vi "写入多个寄存器新.vi"(7 "VISA Resource":refnum<visa-resource-name>, 8 "Error in":errorcluster caption="Error in (no error)", 10 "values":u16[](array[numeric]), 11 "starting address":u16) -> (0 "error out":errorcluster)   [LabVIEW 2016, in "斯坦道CODMn.lvlib"]
uses:
  <vilib>/Plasmionique/MB Master/MB_Master_Serial/MB_Master_Serial.lvclass
  F:/Program Files/National Instruments/LabVIEW 2016/vi.lib/Plasmionique/MB Master/MB_Master/MB_Master.lvclass
  <vilib>/Plasmionique/MB Master/MB Master.lvlib
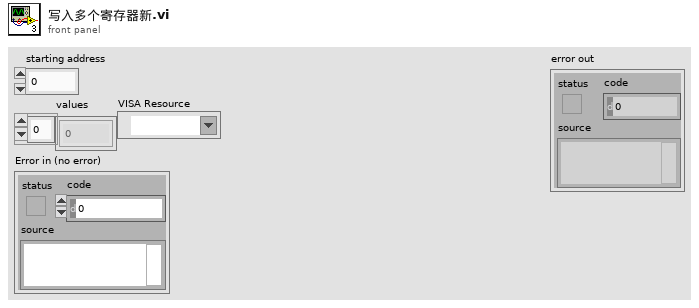
[diagram p1: front panel]
types:
  T1 = cluster{"baud rate (bps)":u32, "stop bits":u16, "parity":u16, "flow control":u16, "timeout":u32, "retries":i32}
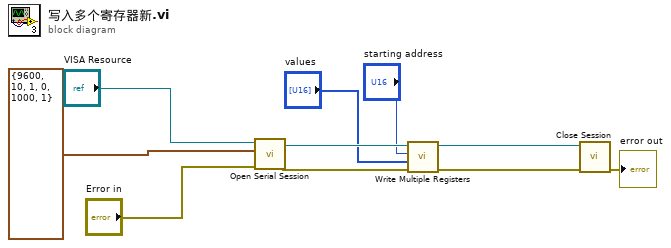
[diagram p0: block diagram]
diagram:
  n1 = call <vilib>:"Open Serial Session.vi"("Error in"="Error in", "Serial Config"=T1 {"baud rate (bps)"=9600, "stop bits"=10, "parity"=1, "flow control"=0, "timeout"=1000, "retries"=1}, "VISA Resource"="VISA Resource") -> ("Error out"=w4:errorcluster, "MB_Serial session"=w10:refnum<class "MB_Master_Serial.lvclass">)  [unwired: 7 in]
  n2 = call <vilib>:"Write Multiple Registers.vi"("error in (no error)"=w4, "values"="values", "starting address"="starting address", "MB session in"=w10) -> ("error out"=w6:errorcluster, "MB session out"=w7:refnum<class "MB_Master_Serial.lvclass">)  [unwired: 6 in]
  n3 = call-dynamic "Close Session.vi"("error in (no error)"=w6, "MB_Serial session"=w7) -> ("error out"=→"error out":errorcluster)  [unwired: 9 in]
